vi "Set Cell (Timestamp).vi"(6 "Column":i32, 7 "Value":timestamp, 8 "error in (no error)":errorcluster, 9 "Row":i32, 10 "Sheet Reference":refnum<k24>) -> (0 "error out":errorcluster, 2 "Sheet Reference out":refnum<k24>)   [LabVIEW 2014]
uses:
  C:/PhaeronGit/LVNPOI/Resources/NPOI 2.1.1 dotnet2/NPOI.dll
  Resources/NPOI 2.1.1 dotnet2/NPOI.dll
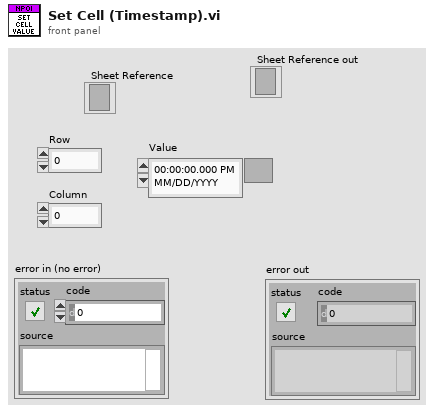
[diagram p1: front panel]
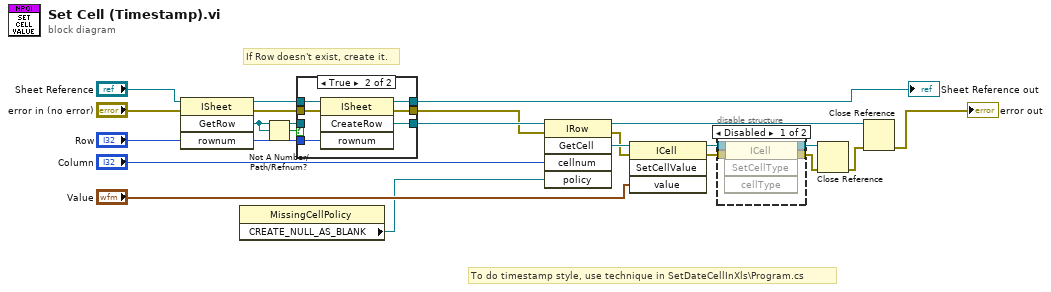
[diagram p0: block diagram]
diagram:
  # "To do timestamp style, use technique in SetDateCellInXls\\Program.cs"
  # "If Row doesn't exist, create it."
  n1 = invoke class="ISheet" method="GetRow"(reference="Sheet Reference", error in="error in (no error)", "rownum"="Row") -> (reference out=w11:refnum<k24>, error out=w12:errorcluster, "GetRow"=w14:refnum<k24>)  [unwired: 1 in, 1 out]
  n2 = property class="MissingCellPolicy"() -> ("CREATE_NULL_AS_BLANK"=w7:refnum<k24>)  [unwired: 2 in, 2 out]
  n3 = Not A Number/Path/Refnum?(number/path/refnum=w14) -> (NaN/Path/Refnum?=w13:bool)
  n4 = case shown="True" w13 {
    tunnel: w11 -> [w25 w31]
    tunnel: w12 -> [w24 w30]
    tunnel: [w24 w29] -> w4
    tunnel: [w25 w28] -> w6
    tunnel: "Row" -> [_ w27]
    tunnel: [w23 w26] -> w5
    tunnel: w14 -> [w23 _]
    frame False {
    }
    frame True {
      n5 = invoke class="ISheet" method="CreateRow"(reference=w31, error in=w30, "rownum"=w27) -> (reference out=w28:refnum<k24>, error out=w29:errorcluster, "CreateRow"=w26:refnum<k24>)  [unwired: 1 in, 1 out]
    }
  }
  "Sheet Reference out" <- w6
  n6 = invoke class="IRow" method="GetCell"(reference=w5, error in=w4, "cellnum"="Column", "policy"=w7) -> (reference out=w22:refnum<k24>, error out=w19:errorcluster, "GetCell"=w20:refnum<k24>)  [unwired: 1 in, 2 out]
  n7 = invoke class="ICell" method="SetCellValue"(reference=w20, error in=w19, "value"="Value") -> (reference out=w2:refnum<k24>, error out=w18:errorcluster)  [unwired: 1 in, 2 out]
  n8 = disable-structure shown="Disabled" {
    disable-tunnel: w18 -> [w35 w36]
    disable-tunnel: [w34 w36] -> w3
    disable-tunnel: w2 -> [w33 w37]
    disable-tunnel: [w32 w37] -> w1
    frame Disabled {
      n9 = invoke class="ICell" method="SetCellType"(reference=w33, error in=w35) -> (reference out=w32:refnum<k24>, error out=w34:errorcluster)  [unwired: 2 in, 2 out]
    }
    frame Enabled {
    }
  }
  n10 = Close Reference(reference=w1, error in (no error)=w3) -> (error out=w17:errorcluster)
  n11 = Close Reference(reference=w22, error in (no error)=w17) -> (error out=→"error out":errorcluster)
